vi "Alerte_Temperature (Sub).vi"(8 "error in (no error)":errorcluster, 9 "Temp Min":dbl, 10 "Temp Max":dbl, 11 "Temp":dbl) -> (1 "error out":errorcluster, 2 "Message d'Alerte":string, 3 "Avertissement?":bool)   [LabVIEW 2018]
doc: "VI qui affiche des alertes (warnings) de température dans une station de météo. Ce VI est une partie du projet de Station Météo de Température, étudié durant la majorité des séances de TP."
panel:
  # "TP N°2"
  # "Mekni Marwen 2ème Année Génie Electrique"
  # "Creation d'Icon Test"
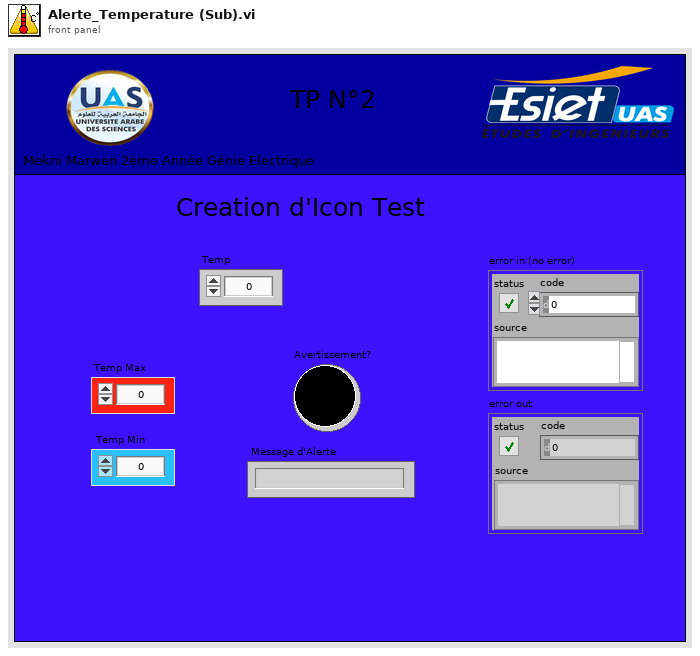
[diagram p1: front panel]
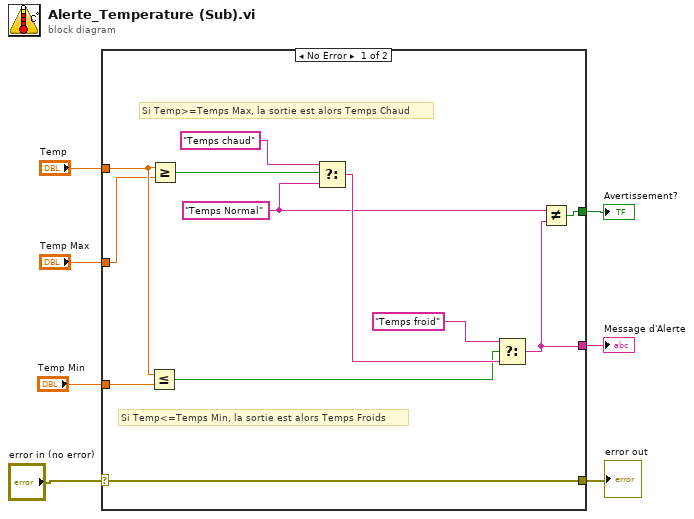
[diagram p0: block diagram]
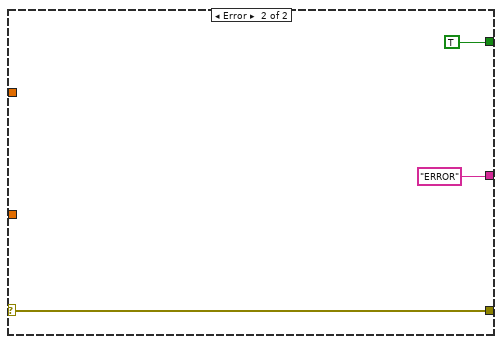
[diagram p2: hidden frame]
diagram:
  n1 = case shown="No Error" "error in (no error)" {
    selector: "error in (no error)" -> [w9 w22]
    tunnel: "Temp Min" -> [w19 _]
    tunnel: "Temp" -> [w18 _]
    tunnel: [w11 TRUE] -> w5
    tunnel: [w10 "ERROR"] -> w4
    tunnel: [w9 w22] -> w2
    tunnel: "Temp Max" -> [w8 _]
    frame No Error {
      w12 = "Temps Normal"
      # "Si Temp>=Temps Max, la sortie est alors Temps Chaud"
      # "Si Temp<=Temps Min, la sortie est alors Temps Froids"
      n2 = Less Or Equal?(x=w18, y=w19) -> (x <= y?=w13:bool)
      n3 = Greater Or Equal?(x=w18, y=w8) -> (x >= y?=w17:bool)
      n4 = Select(t="Temps chaud", s=w17, f=w12) -> (s? t:f=w15:string)
      n5 = Select(t="Temps froid", s=w13, f=w15) -> (s? t:f=w10:string)
      n6 = Not Equal?(x=w12, y=w10) -> (x != y?=w11:bool)
    }
    frame Error {
    }
  }
  "Avertissement?" <- w5
  "Message d'Alerte" <- w4
  "error out" <- w2
